vi "getAnyBuffer.vi"(8 "error in":errorcluster, 10 "buffer size":u64, 11 "Buffers":T1[](array[typedef])) -> (0 "error out":errorcluster, 1 "is locked":bool, 2 "output buffer":T1, 3 "output buffers":T1[](array[typedef]), 5 "index":i32)   [LabVIEW 2016]
uses:
  private/vis/BufferStruct.ctl
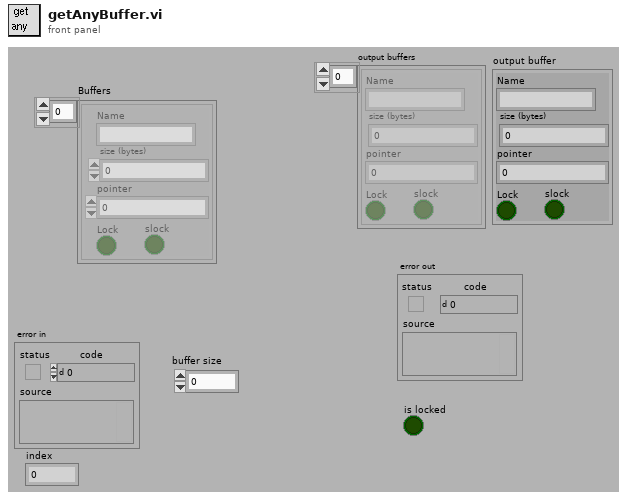
[diagram p1: front panel]
types:
  T1 = typedef "BufferStruct.ctl" = cluster{"Name":string, "size (bytes)":u64, "pointer":u64, "Lock":bool, "slock":bool}
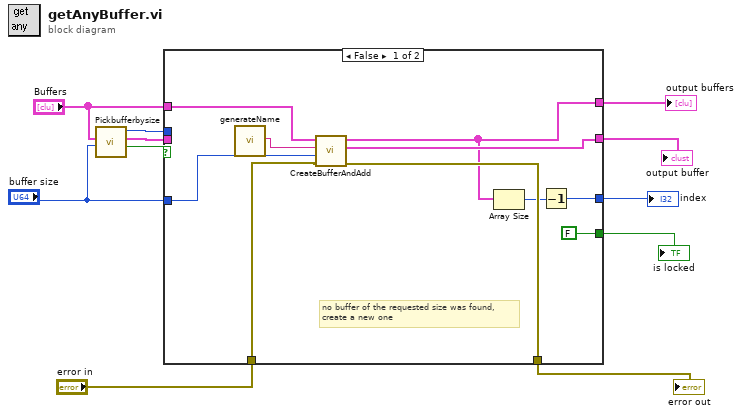
[diagram p0: block diagram]
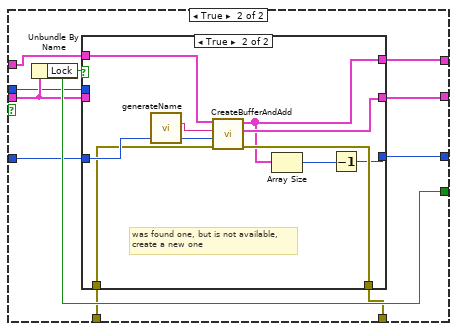
[diagram p2: hidden frame]
diagram:
  n1 = call "Pickbufferbysize.vi"("buffer size"="buffer size", "Buffers"="Buffers") -> ("found"=w11:bool, "buffer found"=w10:T1, "index"=w2:i32)  [unwired: 7 out]
  n2 = case shown="False" w11 {
    tunnel: w10 -> [_ w30]
    tunnel: [w17 w29] -> w9
    tunnel: "buffer size" -> [w21 w26]
    tunnel: "error in" -> [w20 w25]
    tunnel: [w19 w24] -> w8
    tunnel: "Buffers" -> [w18 w28]
    tunnel: [w15 w27] -> w7
    tunnel: [FALSE ("Lock") w31] -> w6
    tunnel: w2 -> [_ w23]
    tunnel: [w13 w22] -> w1
    frame False {
      # "no buffer of the requested size was found,\ncreate a new one"
      n3 = call "generateName.vi"() -> ("buffername"=w12:string)  [unwired: 10 out]
      n4 = call "CreateBufferAndAdd.vi"("error in (no error)"=w20, "Size in Bytes"=w21, "Buffer Name"=w12, "Buffers"=w18) -> ("error out"=w19:errorcluster, "output buffer"=w17:T1, "output buffers"=w15:T1[])  [unwired: 5 out]
      n5 = Array Size(array=w15) -> (size(s)=w14:i32)
      n6 = Decrement(x=w14) -> (x-1=w13:i32)
    }
    frame True {
      n7 = Unbundle By Name(w30) -> ("Lock"=w31:bool)
      n8 = case shown="True" w31 {
        tunnel: w30 -> [w35 _]
        tunnel: [w35 w43] -> w29
        tunnel: w28 -> [w34 w44]
        tunnel: [w34 w39] -> w27
        tunnel: w26 -> [_ w42]
        tunnel: w25 -> [w33 w41]
        tunnel: [w33 w40] -> w24
        tunnel: w23 -> [w32 _]
        tunnel: [w32 w37] -> w22
        frame False {
          # "was found a buffer\navailable"
        }
        frame True {
          # "was found one, but is not available,\ncreate a new one"
          n9 = call "generateName.vi"() -> ("buffername"=w36:string)  [unwired: 10 out]
          n10 = call "CreateBufferAndAdd.vi"("error in (no error)"=w41, "Size in Bytes"=w42, "Buffer Name"=w36, "Buffers"=w44) -> ("error out"=w40:errorcluster, "output buffer"=w43:T1, "output buffers"=w39:T1[])  [unwired: 5 out]
          n11 = Array Size(array=w39) -> (size(s)=w38:i32)
          n12 = Decrement(x=w38) -> (x-1=w37:i32)
        }
      }
    }
  }
  "error out" <- w8
  "output buffers" <- w7
  "output buffer" <- w9
  "is locked" <- w6
  "index" <- w1
